vi "Dequeue Timed Out.vi"(4 "priority in":i32, 6 "timed out?":bool, 7 "Wait Prior":refnum<queue>, 8 "error in (no error)":errorcluster, 9 "element in":refnum<class "Message.lvclass">, 10 "wait queue":refnum<queue>, 11 "priority queue":refnum<data-value>) -> (0 "error out":errorcluster, 1 "priority out":i32, 2 "element out":refnum<class "Message.lvclass">, 3 "really timed out?":bool)   [LabVIEW 2017, in "Actor Framework.lvlib" / "Message Priority Queue.lvclass"]
uses:
  <vilib>/ActorFramework/Message Priority Queue/Message Priority Queue.lvclass
  <vilib>/ActorFramework/Message Priority Queue/DVR Contents.ctl
  <vilib>/ActorFramework/Message/Message.lvclass
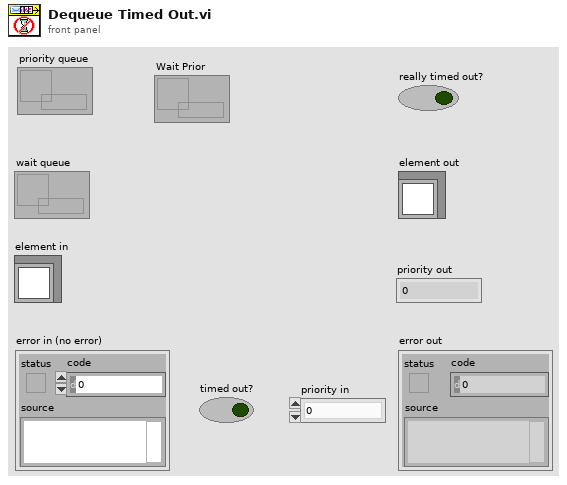
[diagram p1: front panel]
types:
  T1 = typedef "Actor Framework.lvlib/Message Priority Queue.lvclass/DVR Contents.ctl" = cluster{"# Waiting":u32, "Buffers":refnum<queue>[], "Wait Msg":refnum<queue>, "Wait Prior":refnum<queue>}
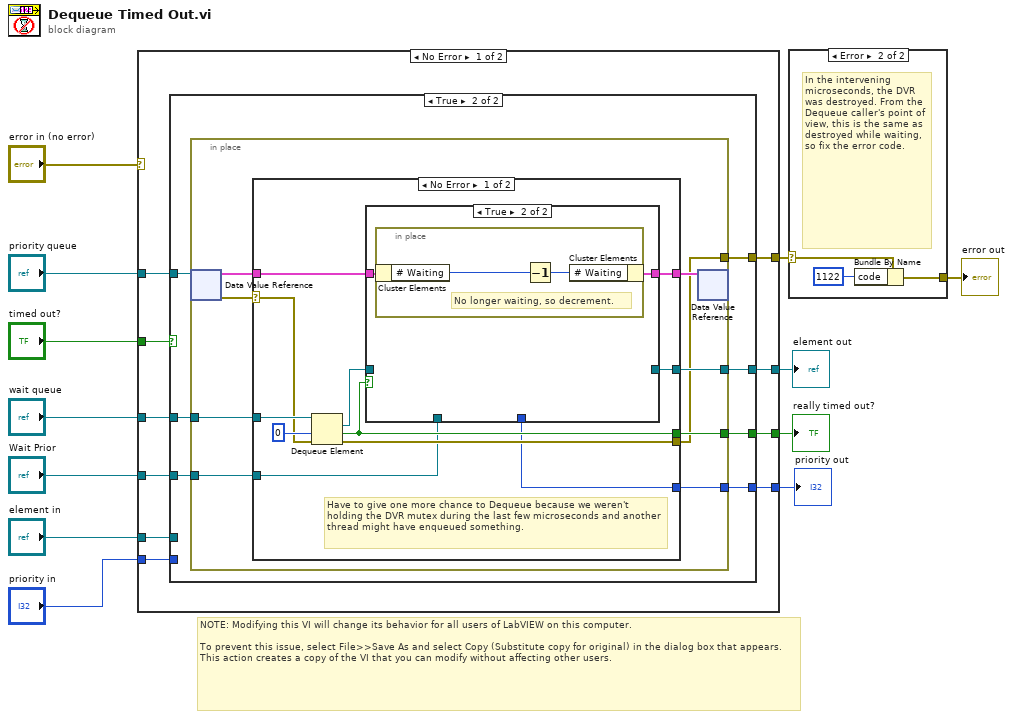
[diagram p0: block diagram]
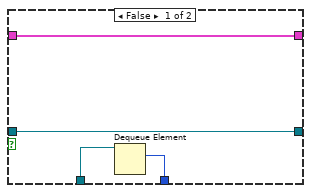
[diagram p4: hidden frame]
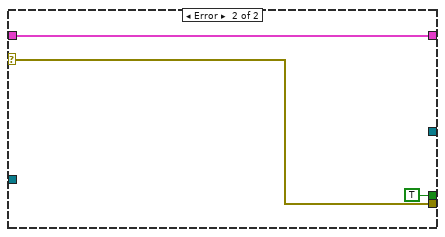
[diagram p5: hidden frame]
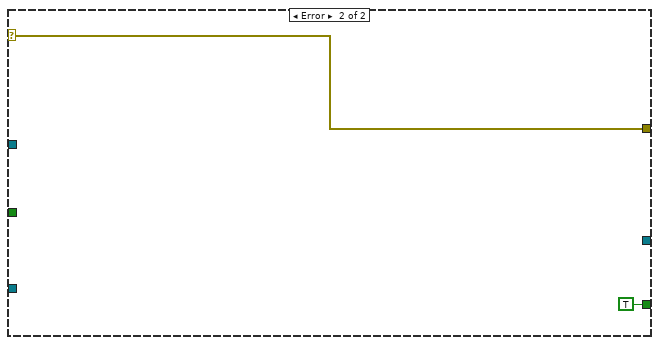
[diagram p6: hidden frame]
diagram:
  # "NOTE: Modifying this VI will change its behavior for all users of LabVIEW on this computer.\n\nTo prevent this issue, select File>>Save As and select Copy (Substitute copy for original) in the dialog box that appears. This action creates a copy of the VI that you can modify without affecting other users."
  n1 = case shown="No Error" "error in (no error)" {
    selector: "error in (no error)" -> [_ w65]
    tunnel: "priority queue" -> [w22 _]
    tunnel: [w21 _] -> w11
    tunnel: "element in" -> [w20 _]
    tunnel: "wait queue" -> [w19 _]
    tunnel: [w18 TRUE ("timed out?")] -> w9
    tunnel: "timed out?" -> [w17 _]
    tunnel: [w16 w65] -> w6
    tunnel: "Wait Prior" -> [w15 _]
    tunnel: [w14 _] -> w2
    tunnel: "priority in" -> [w13 _]
    frame No Error {
      n2 = case shown="True" w17 {
        selector: w17 -> [w25 _]
        tunnel: [w25 w30] -> w18
        tunnel: w19 -> [_ w31]
        tunnel: w20 -> [w24 _]
        tunnel: [w24 w29] -> w21
        tunnel: w22 -> [_ w32]
        tunnel: [_ w28] -> w16
        tunnel: w15 -> [_ w27]
        tunnel: [w23 w26] -> w14
        tunnel: w13 -> [w23 _]
        frame False {
        }
        frame True {
          n3 = in-place {
            in-place-border: w31 -> [w41]
            in-place-border: [w40] -> w30
            in-place-border: [w37] -> w29
            in-place-border: [w35] -> w28
            in-place-border: w27 -> [w34]
            in-place-border: [w33] -> w26
            n4 = in-place-dvr #1(w32) -> (w38:T1, w36:errorcluster)
            n5 = case shown="No Error" w36 {
              selector: w36 -> [w45 w61]
              tunnel: w41 -> [w52 _]
              tunnel: [w50 TRUE ("timed out?")] -> w40
              tunnel: [w49 w63] -> w39
              tunnel: w38 -> [w48 w63]
              tunnel: [w47 _] -> w37
              tunnel: [w44 w61] -> w35
              tunnel: w34 -> [w43 _]
              tunnel: [w42 _] -> w33
              frame No Error {
                # "Have to give one more chance to Dequeue because we weren't holding the DVR mutex during the last few microseconds and another thread might have enqueued something."
                n6 = Dequeue Element(queue=w52, timeout in ms (-1)=0, error in (no error)=w45) -> (element=w46:refnum<class "Message.lvclass">, timed out?=w50:bool, error out=w44:errorcluster)  [unwired: 1 out]
                n7 = case shown="True" w50 {
                  tunnel: [w56 w57] -> w49
                  tunnel: w48 -> [w56 w58]
                  tunnel: [w55 _] -> w47
                  tunnel: w46 -> [w55 _]
                  tunnel: w43 -> [w54 _]
                  tunnel: [w53 _] -> w42
                  frame False {
                    n8 = Dequeue Element(queue=w54) -> (element=w53:i32)  [unwired: 2 in, 3 out]
                  }
                  frame True {
                    n9 = in-place {
                      # "No longer waiting, so decrement."
                      n10 = in-place-cluster #2(w58) -> ("# Waiting"=w60:u32)
                      n11 = Decrement(x=w60) -> (x-1=w59:u32)
                      n12 = in-place-cluster #2("# Waiting"=w59) -> (w57:T1)
                    }
                  }
                }
              }
              frame Error {
              }
            }
            n13 = in-place-dvr #1(w39) -> ()  [unwired: 2 out]
          }
        }
      }
    }
    frame Error {
    }
  }
  "element out" <- w11
  "really timed out?" <- w9
  "priority out" <- w2
  n14 = case shown="Error" w6 {
    selector: w6 -> [w66 w67]
    tunnel: [w66 w68] -> w7
    frame No Error {
    }
    frame Error {
      # "In the intervening microseconds, the DVR was destroyed. From the Dequeue caller's point of view, this is the same as destroyed while waiting, so fix the error code."
      n15 = Bundle By Name(cluster=w67, "code"=1122) -> (w68:errorcluster)
    }
  }
  "error out" <- w7
